vi "_s_Bronkhorst Serial Change Setpoint.vi"(5 "Auto":bool, 7 "Comunicaciones":T1={"Flujo_1"="ASRL6::INSTR", "Brk1"=FALSE, "Flujo_2"="ASRL6::INSTR", "Brk2"=FALSE, "Flujo_3"="ASRL6::INSTR", "Brk3"=FALSE, "Flujo_4"="ASRL6::INSTR", "Brk4"=FALSE, "Eurothe"="ASRL6::INSTR", "Eurot"=FALSE, "Balanza"="ASRL6::INSTR", "Bal"=FALSE, "eValPos"="ASRL6::INSTR", "eVal"=FALSE, "flowbus"="ASRL6::INSTR", "fb"=FALSE}, 8 "error in (no error)":errorcluster, 9 "Nuevo Setpoint":dbl caption="asd" format="%.2f", 10 "Dispositivos":T2=[["3", "NO", "M0000013", "Air", "1", "ln/mn", "0", "0"], ["4", "NO", "M0000014", "Air", "1", "ln/mn", "0", "0"], ["5", "NO", "M0000015", "Air", "1", "ln/mn", "0", "0"], ["6", "NO", "M0000016", "Air", "1", "ln/mn", "0", "0"], ["7", "NO", "M0000017", "Air", "1", "ln/mn", "0", "0"], ["8", "NO", "M0000018", "Air", "1", "ln/mn", "0", "0"], ["9", "NO", "M0000019", "Air", "1", "ln/mn", "0", "0"], ["10", "NO", "M0000020", "Air", "1", "ln/mn", "0", "0"], ["11", "NO", "M0000021", "Air", "1", "ln/mn", "0", "0"]] caption="MassFlowControllers", 11 "Address":i32) -> (0 "error out":errorcluster, 1 "Nuevo Setpoint 2":dbl caption="asd" format="%#g")   [LabVIEW 2013]
uses:
  _s_TablaBronkhorst.ctl
  Controles/P2018 Com Control.ctl
  _s_Bronkhorst Control.ctl
panel:
  out "Error":bool
  out "Activo":string caption="asd"
  out "Actual Setpoint":dbl caption="asd" format="%.2f"
  out "Com":string caption="asd"
  out "Units":string caption="asd"
  out "Rango max":string caption="asd"
  out "Rango min":string caption="asd"
  out "Gas":string caption="asd"
  out "Serial Number":string caption="asd"
  in  "Cancel":bool
  in  "OK2":bool
  # "Cambio en setpoint"
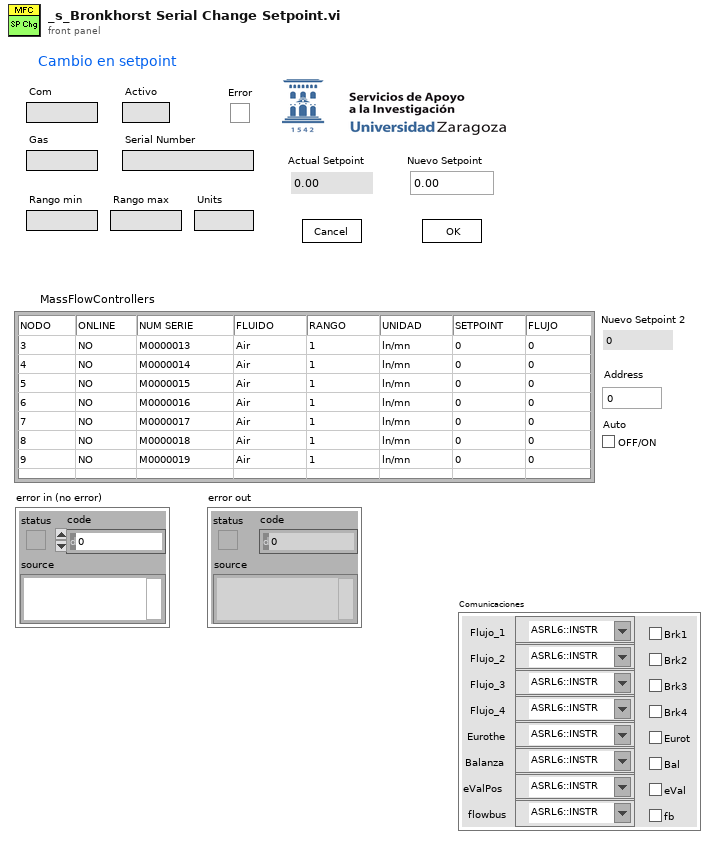
[diagram p1: front panel]
types:
  T1 = typedef "P2018 Com Control.ctl" = cluster{"Flujo_1":refnum<visa-resource-name>, "Brk1":bool, "Flujo_2":refnum<visa-resource-name>, "Brk2":bool, "Flujo_3":refnum<visa-resource-name>, "Brk3":bool, "Flujo_4":refnum<visa-resource-name>, "Brk4":bool, "Eurothe":refnum<visa-resource-name>, "Eurot":bool, "Balanza":refnum<visa-resource-name>, "Bal":bool, "eValPos":refnum<visa-resource-name>, "eVal":bool, "flowbus":refnum<visa-resource-name>, "fb":bool}
  T2 = typedef "_s_TablaBronkhorst.ctl" = string[][]
  T3 = typedef "_s_Bronkhorst Control.ctl" = enum16{"Inicializar", "Request IdnString", "Request Serial Number", "Request Fluid Number", "Request Fluid Name", "Request Sensor Type", "Request Cap 0", "Request Cap100", "Request Units", "Request CapUnitStr", "Request Setpoint %", "Request Setpoint", "Request Measure %", "Request Measure ", "Send Control Mode", "Send Fluid Number", "Send Setpoint %", "Send Setpoint", "Shutdown"}
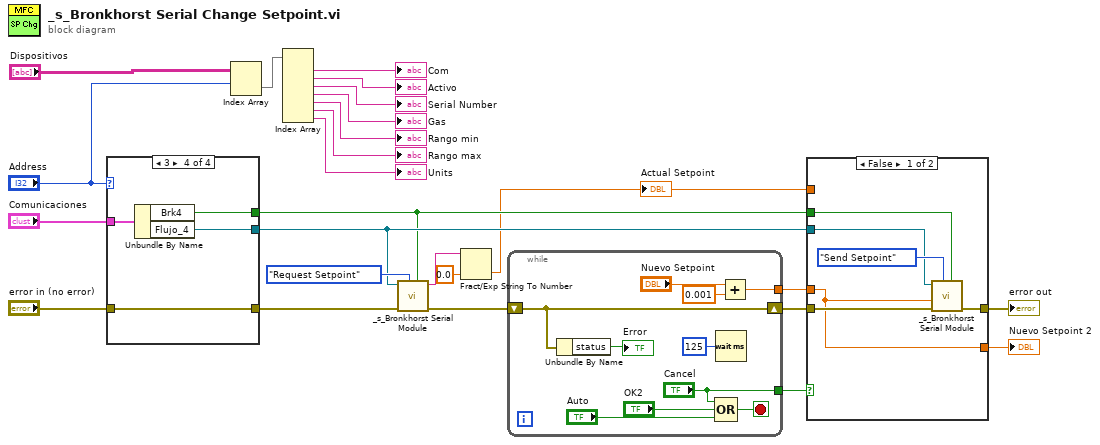
[diagram p0: block diagram]
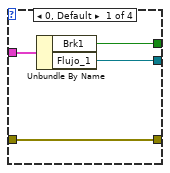
[diagram p2: hidden frame]
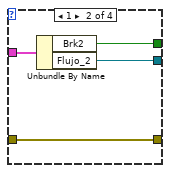
[diagram p3: hidden frame]
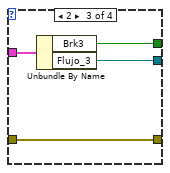
[diagram p4: hidden frame]
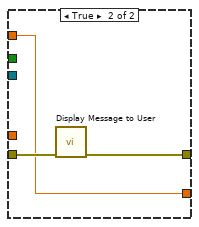
[diagram p5: hidden frame]
diagram:
  n1 = case shown="3" "Address" {
    tunnel: "error in (no error)" -> [w27 w31 w35 w39]
    tunnel: "Comunicaciones" -> [w29 w33 w37 w41]
    tunnel: [w28 w32 w36 w40] -> w4
    tunnel: [w27 w31 w35 w39] -> w6
    tunnel: [w26 w30 w34 w38] -> w5
    frame 0, Default {
      n2 = Unbundle By Name(w29) -> ("Brk1"=w28:bool, "Flujo_1"=w26:refnum<visa-resource-name>)
    }
    frame 1 {
      n3 = Unbundle By Name(w33) -> ("Brk2"=w32:bool, "Flujo_2"=w30:refnum<visa-resource-name>)
    }
    frame 2 {
      n4 = Unbundle By Name(w37) -> ("Brk3"=w36:bool, "Flujo_3"=w34:refnum<visa-resource-name>)
    }
    frame 3 {
      n5 = Unbundle By Name(w41) -> ("Brk4"=w40:bool, "Flujo_4"=w38:refnum<visa-resource-name>)
    }
  }
  n6 = Index Array(array="Dispositivos", index (row)="Address") -> (element=w21:string[])  [unwired: 1 in]
  n7 = Index Array(array=w21) -> (element #1=→"Com":string, element #2=→"Activo":string, element #3=→"Serial Number":string, element #4=→"Gas":string, element #5=→"Rango min":string, element #6=→"Rango max":string, element #7=→"Units":string)  [unwired: 7 in]
  n8 = call "_s_Bronkhorst Serial Module.vi"("Module (T:Enable)"=w4, "Command"=_s_Bronkhorst_Control."Request Setpoint", "error in (no error)"=w6, "VISA resource name"=w5) -> ("error out"=w7:errorcluster, "Value"=w8:string)  [unwired: 4 in, 2 out]
  n9 = Fract/Exp String To Number(string=w8, default (0 dbl)=0.0 ("default (0 DBL)")) -> (number=w3:dbl)  [unwired: 2 in, 1 out]
  "Actual Setpoint" <- w3
  n10 = while {
    shift-right: [w45] -> w16
    shift-left: w7 -> [w45]
    tunnel: ["Cancel"] -> w17
    tunnel: [w44] -> w12
    stop <- w50 stop-if-true
    n11 = Unbundle By Name(w45) -> ("status"=→"Error":bool)
    n12 = Compound Arithmetic op=OR("Cancel", "OK2", "Auto") -> (w50:bool)
    n13 = Wait (ms)(milliseconds to wait=u32 125) -> ()  [unwired: 1 out]
    n14 = Add(x="Nuevo Setpoint", y=0.001) -> (x+y=w44:dbl)
  }
  n15 = case shown="False" w17 {
    tunnel: w16 -> [w57 w60]
    tunnel: [w56 w59] -> w15
    tunnel: w12 -> [w52 _]
    tunnel: w5 -> [w54 _]
    tunnel: w4 -> [w53 _]
    tunnel: w3 -> [_ w58]
    tunnel: [w52 w58] -> w2
    frame False {
      n16 = call "_s_Bronkhorst Serial Module.vi"("Module (T:Enable)"=w53, "Command"=_s_Bronkhorst_Control."Send Setpoint", "error in (no error)"=w57, "Setpoint %"=w52, "VISA resource name"=w54) -> ("error out"=w56:errorcluster)  [unwired: 3 in, 3 out]
    }
    frame True {
      n17 = call "Display Message to User"("error in (no error)"=w60) -> ("error out"=w59:errorcluster)  [unwired: 9 in, 1 out]
    }
  }
  "error out" <- w15
  "Nuevo Setpoint 2" <- w2
